vi "Write Tactics.vi"(8 "error in (no error)":errorcluster, 10 "Tactics":T1, 11 "PrimaryAttackerRole_v2 in":refnum<class "PrimaryAttackerRole_v2.lvclass">) -> (0 "error out":errorcluster, 3 "PrimaryAttackerRole_v2 out":refnum<class "PrimaryAttackerRole_v2.lvclass">)   [LabVIEW 2023, in "PrimaryAttackerRole_v2.lvclass"]
uses:
  PrimaryAttackerRole_v2.lvclass
  Tactics/InterceptBallTactic_v2_class/InterceptBallTactic_v2.lvclass
  PrimaryAttackerRole_v2.lvclass/PrimaryAttackerRole_v2.ctl
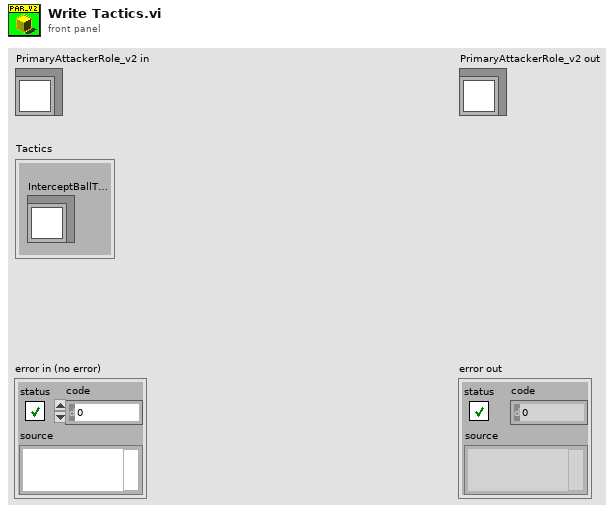
[diagram p1: front panel]
types:
  T1 = cluster{"InterceptBallTactic_v2":refnum<class "InterceptBallTactic_v2.lvclass">}
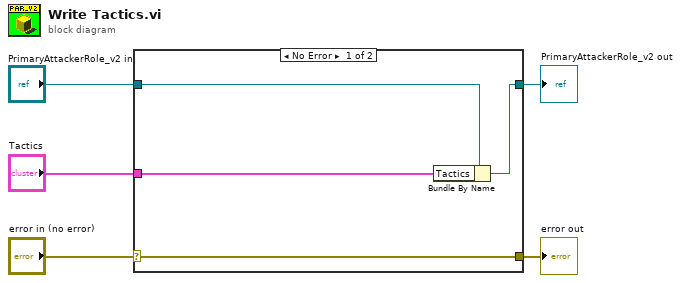
[diagram p0: block diagram]
diagram:
  n1 = case shown="No Error" "error in (no error)" {
    selector: "error in (no error)" -> [w9 w10]
    tunnel: [w9 w10] -> w4
    tunnel: [w7 w11] -> w2
    tunnel: "PrimaryAttackerRole_v2 in" -> [w8 w11]
    tunnel: "Tactics" -> [w6 _]
    frame No Error {
      n2 = Bundle By Name(cluster=w8, "Tactics"=w6) -> (w7:refnum<class "PrimaryAttackerRole_v2.lvclass">)
    }
    frame Error {
    }
  }
  "error out" <- w4
  "PrimaryAttackerRole_v2 out" <- w2
